vi "OnDataChange.vi"(0 "OxxiusLaserController in":refnum<class "OxxiusLaserController.lvclass">, 1 "DataExchange":T1, 3 "error in (no error)":errorcluster) -> (7 "OxxiusLaserController out":refnum<class "OxxiusLaserController.lvclass">, 10 "error out":errorcluster)   [LabVIEW 2020, in "OxxiusLaserController.lvlib" / "OxxiusLaserController.lvclass"]
uses:
  OxxiusLaserController.lvclass
  Model/Hardware Abstraction Layer/Component/Device/Device/DataExchange.ctl
  Interface/DataListener/DataListener.lvclass
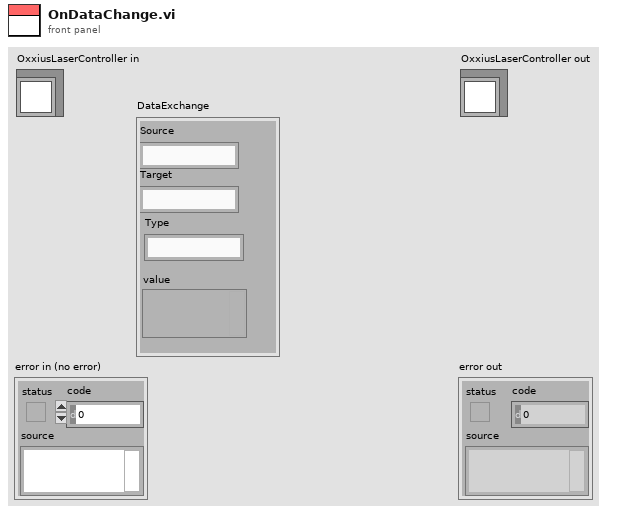
[diagram p1: front panel]
types:
  T1 = typedef "DataListener.lvclass/DataExchange.ctl" = cluster{"Source":string, "Target":string, "Type":string, "value":variant}
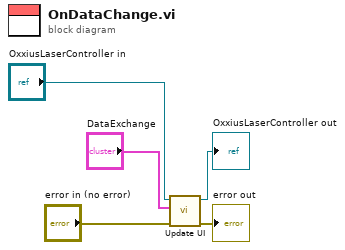
[diagram p0: block diagram]
diagram:
  n1 = call-dynamic "Update UI.vi"("error in (no error)"="error in (no error)", "DataExchange"="DataExchange", "Laser Oxxius Controller in"="OxxiusLaserController in") -> ("error out"=→"error out":errorcluster, "Laser Oxxius Controller out"=→"OxxiusLaserController out":refnum<class "OxxiusLaserController.lvclass">)  [unwired: 7 in]
